vi "Get state DSP402.vi"(1 "DSP402 in":refnum<class "DSP402.lvclass">) -> (0 "State":T1)   [LabVIEW 2017, in "canopen.lvlib" / "DSP402.lvclass"]
uses:
  DSP402.lvclass
  DriveState.ctl
  DSP402.lvclass/DSP402.ctl
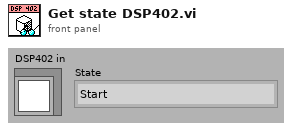
[diagram p1: front panel]
types:
  T1 = typedef "canopen.lvlib/DSP402.lvclass/DriveState.ctl" = enum16{"Start", "Not ready to switch on", "Switch on disabled", "Ready to switch on", "Switched on", "Operation enable", "Fault reaction active", "Fault", "Quick stop active"}
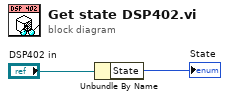
[diagram p0: block diagram]
diagram:
  n1 = Unbundle By Name("DSP402 in") -> ("State"=→"State":T1)
